vi "Direction to Motor Controller.vi"(5 "Turn Percent Limit":dbl, 7 "Percent Limit":dbl, 10 "Angular vel (rad/s)":dbl(slide) scale=-2.0..2.0, 11 "Vel (m/s)":dbl(slide) scale=0.0..10.0) -> (1 "Turn Direction":string, 3 "Forward Direction":string)   [LabVIEW 2013]
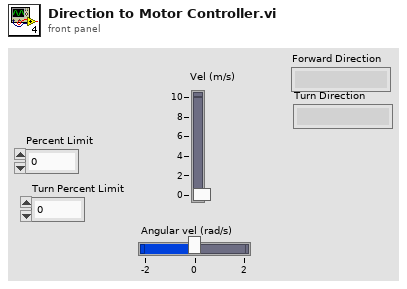
[diagram p1: front panel]
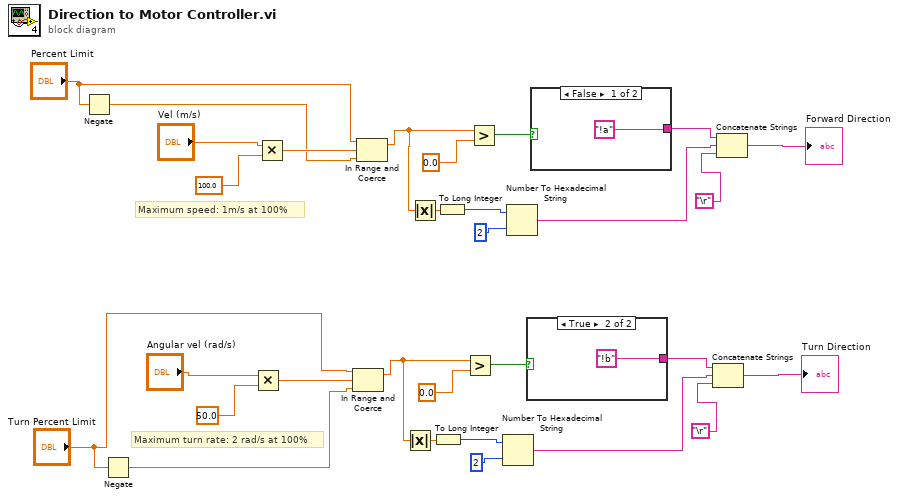
[diagram p0: block diagram]
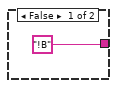
[diagram p2: hidden frame]
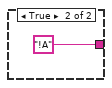
[diagram p3: hidden frame]
diagram:
  # "Maximum turn rate: 2 rad/s at 100%"
  # "Maximum speed: 1m/s at 100%"
  n1 = Negate(x="Percent Limit") -> (-x=w9:dbl)
  n2 = Negate(x="Turn Percent Limit") -> (-x=w3:dbl)
  n3 = Multiply(x="Angular vel (rad/s)", y=50.0) -> (x*y=w19:dbl)
  n4 = Multiply(x="Vel (m/s)", y=100.0) -> (x*y=w28:dbl)
  n5 = In Range and Coerce(upper limit="Turn Percent Limit", x=w19, lower limit=w3) -> (coerced(x)=w5:dbl)  [unwired: 1 out]
  n6 = In Range and Coerce(upper limit="Percent Limit", x=w28, lower limit=w9) -> (coerced(x)=w1:dbl)  [unwired: 1 out]
  n7 = Absolute Value(x=w5) -> (abs(x)=w6:dbl)
  n8 = Absolute Value(x=w1) -> (abs(x)=w2:dbl)
  n9 = To Long Integer(number=w6) -> (32bit integer=w14:i32)
  n10 = To Long Integer(number=w2) -> (32bit integer=w23:i32)
  n11 = Greater?(x=w5, y=0.0) -> (0:w18:bool)
  n12 = Greater?(x=w1, y=0.0) -> (0:w27:bool)
  n13 = Number To Hexadecimal String(1:i16 2 ("width (-)"), 2:w14) -> (0:w13:string)
  n14 = Number To Hexadecimal String(1:i16 2 ("width (-)"), 2:w23) -> (0:w22:string)
  n15 = case shown="True" w18 {
    tunnel: ["!B" "!b"] -> w16
    frame False {
    }
    frame True {
    }
  }
  n16 = case shown="False" w27 {
    tunnel: ["!a" "!A"] -> w25
    frame False {
    }
    frame True {
    }
  }
  n17 = Concatenate Strings(w16, w13, "\r") -> (→"Turn Direction":string)
  n18 = Concatenate Strings(w25, w22, "\r") -> (→"Forward Direction":string)
